vi "MU Mt Analyze Result Max Offset Error.vi"(8 "error in (no error)":errorcluster, 10 "MtTrackOffset":u8, 11 "MtSync_AnalyzeResultHandle":T1) -> (0 "error out":errorcluster, 3 "MaxOffsetError":dbl)   [LabVIEW 2017, in "MU_3SL_interface.lvlib"]
uses:
  MU_3SL_interface.lvlib
  handles/mtSyncAnalyzeResultHandle.ctl
  lib/MU_3SL_interface.dll
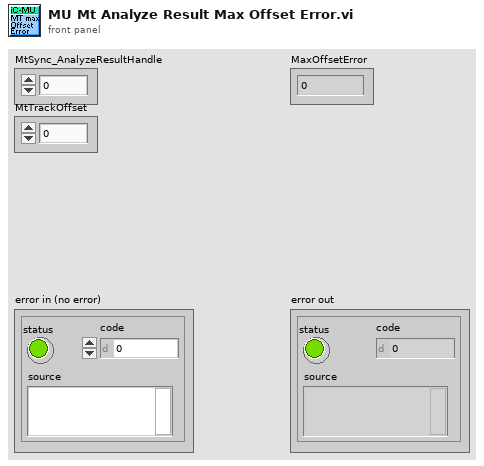
[diagram p1: front panel]
types:
  T1 = typedef "MU_3SL_interface.lvlib/mtSyncAnalyzeResultHandle.ctl" = u64
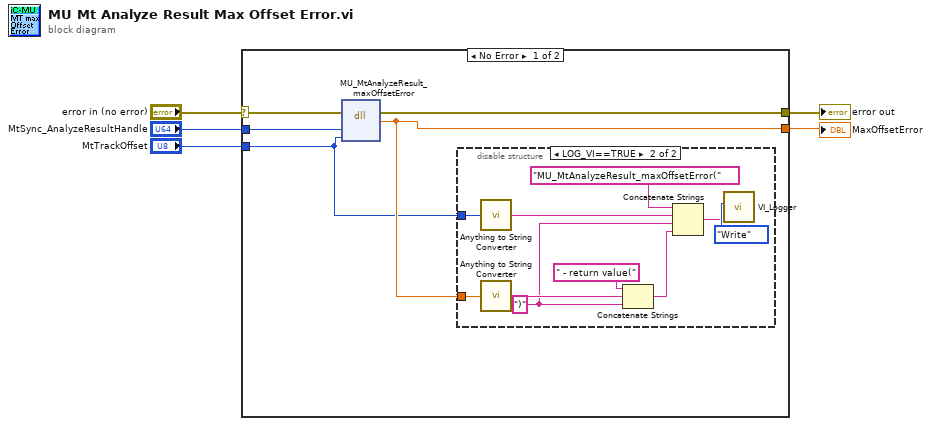
[diagram p0: block diagram]
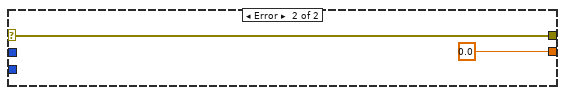
[diagram p3: hidden frame]
diagram:
  n1 = case shown="No Error" "error in (no error)" {
    selector: "error in (no error)" -> [w10 w22]
    tunnel: [w9 0.0 ("Return Value")] -> w2
    tunnel: [w8 w22] -> w5
    tunnel: "MtSync_AnalyzeResultHandle" -> [w7 _]
    tunnel: "MtTrackOffset" -> [w6 _]
    frame No Error {
      n2 = dll-call lib="C:/Users/bes/AppData/Roaming/work/mu_9so/icsubmodules/soft_mu_3sl_master/lv_interface/lib/MU_3SL_interface**.*" fn="MU_MtAnalyzeResult_maxOffsetError"(error in=w10, "MtAnalyzeResultHandle"=w7, "MtTrackOffset"=w6) -> (error out=w8:errorcluster, "MaxOffsetError"=w9:dbl)  [unwired: 4 in, 1 out]
      n3 = disable-structure shown="LOG_VI==TRUE" {
        disable-tunnel: w9 -> [_ w16]
        disable-tunnel: w6 -> [_ w14]
        frame condition #0 {
        }
        frame condition #1 (active) {
          w12 = ")" ("string")
          n4 = call "Anything to String Converter.vi"("anything"=w14) -> ("String"=w13:string)
          n5 = call "Anything to String Converter.vi"("anything"=w16) -> ("String"=w15:string)
          n6 = Concatenate Strings(" - return value(" ("string"), w15, w12) -> (w11:string)
          n7 = Concatenate Strings("MU_MtAnalyzeResult_maxOffsetError(" ("Info in"), w13, w12, w11) -> (w18:string)
          n8 = call "VI_Logger.vi"("Action (Read)"=enum16{"Write", "Read"}."Write", "Info in"=w18) -> ()  [unwired: 8 in, 2 out]
        }
      }
    }
    frame Error {
    }
  }
  "error out" <- w5
  "MaxOffsetError" <- w2
